vi "calculate_path_length.vi"(8 "error in (no error)":errorcluster, 10 "path in":refnum<class "SpaceVector.lvclass">[](array[class])) -> (0 "error out":errorcluster, 2 "length":dbl[unit])   [LabVIEW 2017, in "SpaceVector.lvclass"]
uses:
  SpaceVector.lvclass
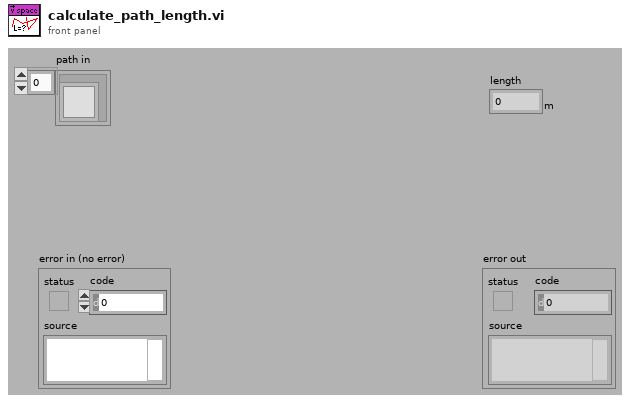
[diagram p1: front panel]
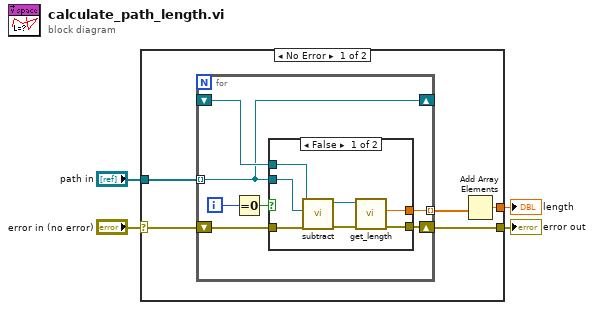
[diagram p0: block diagram]
diagram:
  n1 = case shown="No Error" "error in (no error)" {
    selector: "error in (no error)" -> [w9 w25]
    tunnel: [w8 w25] -> w3
    tunnel: "path in" -> [w7 _]
    tunnel: [w5 _] -> w1
    frame No Error {
      n2 = for {
        shift-right: [w14] -> w8
        shift-left: w9 -> [w16]
        tunnel: w7 -> [w11] mode=indexing
        shift-right: [w11] -> _
        shift-left: _ -> [w15]
        tunnel: [w10] -> w6 mode=indexing
        i -> [w13]
        n3 = Equal To 0?(x=w13) -> (x = 0?=w12:bool)
        n4 = case shown="False" w12 {
          tunnel: w16 -> [w23 w24]
          tunnel: w15 -> [w22 _]
          tunnel: w11 -> [w19 _]
          tunnel: [w18 w24] -> w14
          tunnel: [w17 _] -> w10
          frame False {
            n5 = call "subtract.vi"("error in (no error)"=w23, "subtrahend"=w19, "SpaceVector in"=w22) -> ("error out"=w21:errorcluster, "SpaceVector out"=w20:refnum<class "SpaceVector.lvclass">)  [unwired: 7 in]
            n6 = call "get_length.vi"("error in (no error)"=w21, "SpaceVector in"=w20) -> ("error out"=w18:errorcluster, "length"=w17:dbl[unit])  [unwired: 7 in, 1 out]
          }
          frame True {
          }
        }
      }
      n7 = Add Array Elements(numeric array=w6) -> (sum=w5:dbl[unit])
    }
    frame Error {
    }
  }
  "error out" <- w3
  "length" <- w1
